vi "ControlSpecificValue.vi"(0 "Control in":refnum<vi>, 11 "Error In":errorcluster) -> (4 "Control out":refnum<vi>, 6 "Value":variant, 15 "Error Out":errorcluster)   [LabVIEW 2016, in "Drona.lvlib" / "AssertControlValue.lvlib"]
doc: "Based on the specific control, it result the corresponding value"
uses:
  AssertControlValue.lvlib
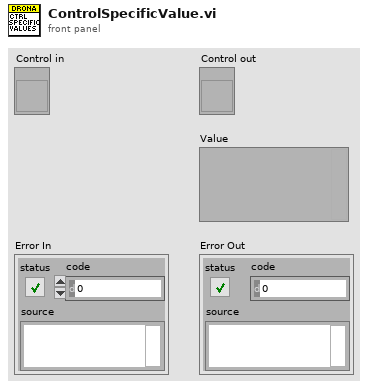
[diagram p1: front panel]
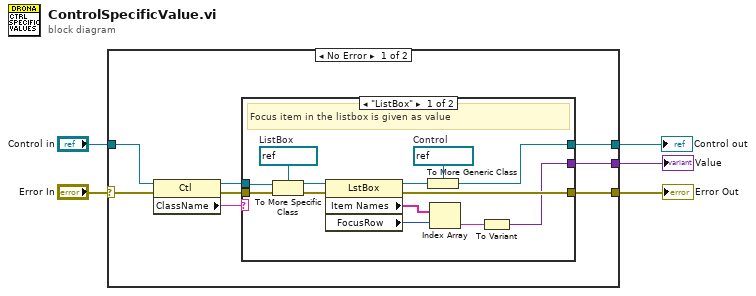
[diagram p0: block diagram]
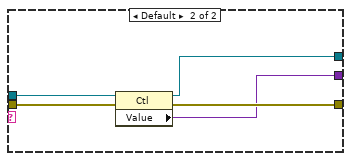
[diagram p2: hidden frame]
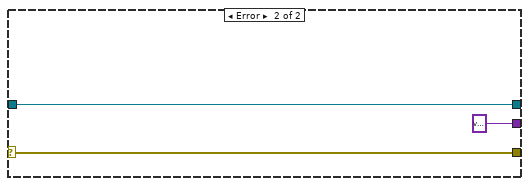
[diagram p3: hidden frame]
diagram:
  n1 = case shown="No Error" "Error In" {
    selector: "Error In" -> [w13 w33]
    tunnel: [w6 w34] -> w5
    tunnel: [w7 variant ("Value")] -> w4
    tunnel: "Control in" -> [w10 w34]
    tunnel: [w12 w33] -> w1
    frame No Error {
      n2 = property class="Ctl"(reference=w10, error in=w13) -> (reference out=w8:refnum<vi>, error out=w11:errorcluster, "ClassName"=w9:string)
      n3 = case shown="\"ListBox\"" w9 {
        tunnel: [w22 w31] -> w12
        tunnel: w11 -> [w26 w30]
        tunnel: w8 -> [w24 w29]
        tunnel: [w14 w28] -> w6
        tunnel: [w17 w27] -> w7
        frame "ListBox" {
          w15 = refnum<vi> refnum  # Control
          w23 = refnum<vi> refnum  # ListBox
          # "Focus item in the listbox is given as value"
          n4 = To More Specific Class(target class=w23, reference=w24, error in=w26) -> (specific class reference=w21:refnum<vi>, error out=w25:errorcluster)
          n5 = property class="LstBox"(reference=w21, error in=w25) -> (reference out=w16:refnum<vi>, error out=w22:errorcluster, "Item Names"=w19:string[], "FocusRow"=w20:i32)
          n6 = To More Generic Class(target class=w15, reference=w16) -> (generic class reference=w14:refnum<vi>)
          n7 = Index Array(array=w19, index=w20) -> (element=w18:string)
          n8 = To Variant(anything=w18) -> (Variant=w17:variant)
        }
        frame Default {
          n9 = property on="Property Node" class="Ctl"(reference=w29, error in=w30) -> (reference out=w28:refnum<vi>, error out=w31:errorcluster, "Value"=w27:variant)
        }
      }
    }
    frame Error {
    }
  }
  "Control out" <- w5
  "Value" <- w4
  "Error Out" <- w1
